vi "Kbd_Event_key_demo(copy).vi"() -> ()   [LabVIEW 2012]
panel:
  in  "error in":errorcluster
  out "error out":errorcluster
  in  "String":string="1234"
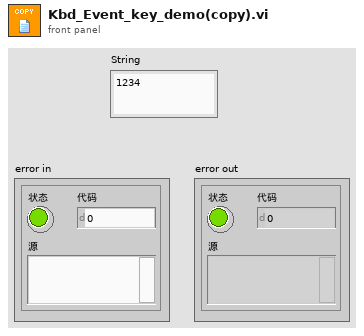
[diagram p1: front panel]
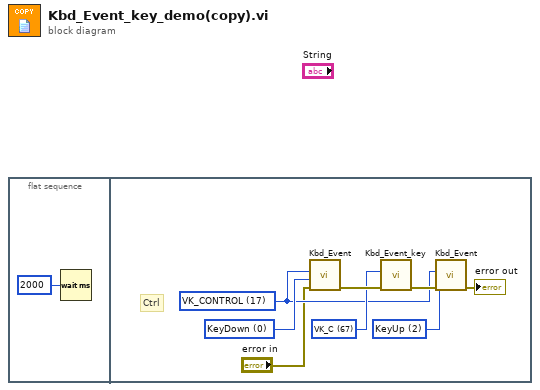
[diagram p0: block diagram]
diagram:
  n1 = flat-sequence {
    frame #0 {
      n2 = Wait (ms)(milliseconds to wait=u32 2000) -> ()  [unwired: 1 out]
    }
    frame #1 {
      w7 = u8 67 items=["Undefined", "VK_LBUTTON", "VK_RBUTTON", "VK_CANCEL", "VK_MBUTTON", "VK_XBUTTON1", "VK_XBUTTON2", "Undefined", "VK_BACK", "VK_TAB", "Reserved", "Reserved", "VK_CLEAR", "VK_RETURN", "Undefined", "Undefined", "VK_SHIFT", "VK_CONTROL", "VK_MENU", "VK_PAUSE", "VK_CAPITAL", "VK_KANA", "Undefined", "VK_JUNJA", "VK_FINAL", "VK_HANJA", "Undefined", "VK_ESCAPE", "VK_CONVERT", "VK_NONCONVERT", "VK_ACCEPT", "VK_MODECHANGE", "VK_SPACE", "VK_PRIOR", "VK_NEXT", "VK_END", "VK_HOME", "VK_LEFT", "VK_UP", "VK_RIGHT", "VK_DOWN", "VK_SELECT", "VK_PRINT", "VK_EXECUTE", "VK_SNAPSHOT", "VK_INSERT", "VK_DELETE", "VK_HELP", "VK_0", "VK_1", "VK_2", "VK_3", "VK_4", "VK_5", "VK_6", "VK_7", "VK_8", "VK_9", "Undefined", "Undefined", "Undefined", "Undefined", "Undefined", "Undefined", "Undefined", "VK_A", "VK_B", "VK_C", "VK_D", "VK_E", "VK_F", "VK_G", "VK_H", "VK_I", "VK_J", "VK_K", "VK_L", "VK_M", "VK_N", "VK_O", "VK_P", "VK_Q", "VK_R", "VK_S", "VK_T", "VK_U", "VK_V", "VK_W", "VK_X", "VK_Y", "VK_Z", "VK_LWIN", "VK_RWIN", "VK_APPS", "Reserved", "VK_SLEEP", "VK_NUMPAD0", "VK_NUMPAD1", "VK_NUMPAD2", "VK_NUMPAD3", "VK_NUMPAD4", "VK_NUMPAD5", "VK_NUMPAD6", "VK_NUMPAD7", "VK_NUMPAD8", "VK_NUMPAD9", "VK_MULTIPLY", "VK_ADD", "VK_SEPARATOR", "VK_SUBTRACT", "VK_DECIMAL", "VK_DIVIDE", "VK_F1", "VK_F2", "VK_F3", "VK_F4", "VK_F5", "VK_F6", "VK_F7", "VK_F8", "VK_F9", "VK_F10", "VK_F11", "VK_F12", "VK_F13", "VK_F14", "VK_F15", "VK_F16", "VK_F17", "VK_F18", "VK_F19  ", "VK_F20 ", "VK_F21", "VK_F22 ", "VK_F23", "VK_F24", "Unsigned", "Unsigned", "Unsigned", "Unsigned", "Unsigned", "Unsigned", "Unsigned", "Unsigned", "VK_NUMLOCK", "VK_SCROLL", "OEM Specific", " OEM Speicfic", "OEM Speicfic", "OEM Specific", "OEM Specific", "Unassigned", "Unassigned", "Unassigned", "Unassigned", "Unassigned", "Unassigned", "Unassigned", "Unassigned", "Unassigned", "VK_LSHIFT", "VK_RSHIFT", "VK_LCONTROL", "VK_RCONTROL", "VK_LMENU", "VK_RMENU", "VK_BROWSER_BACK", "VK_BROWSER_FORWARD", "VK_BROWSER_REFRESH", "VK_BROWSER_STOP", "VK_BROWSER_SEARCH", "VK_BROWSER_FAVORITES ", "VK_BROWSER_HOME", "VK_VOLUME_MUTE", "VK_VOLUME_DOWN", "VK_VOLUME_UP", "VK_MEDIA_NEXT_TRACK", "VK_MEDIA_PREV_TRACK", "VK_MEDIA_STOP ", "VK_MEDIA_PLAY_PAUSE", "VK_LAUNCH_MAIL", "VK_LAUNCH_MEDIA_SELECT", "VK_LAUNCH_APP1", "VK_LAUNCH_APP2", "Reserved", "Reserved", "VK_OEM_1(;:)", "VK_OEM_PLUS(+) ", "VK_OEM_COMMA(,)", "VK_OEM_MINUS(-)", "VK_OEM_PERIOD(.)", "VK_OEM_2(/?)", "VK_OEM_3(~`)", "Reserved", "Reserved", "Reserved", "Reserved", "Reserved", "Reserved", "Reserved", "Reserved", "Reserved", "Reserved", "Reserved", "Reserved", "Reserved", "Reserved", "Reserved", "Reserved", "Reserved", "Reserved", "Reserved", "Reserved", "Reserved", "Reserved", "Reserved", "Reserved", "Reserved", "Reserved", "VK_OEM_4 ([{)", "VK_OEM_5 (\\|)", "VK_OEM_6 (]})", "VK_OEM_7 ('\")", "VK_OEM_8", "Reserved", "Reserved", "VK_OEM_102", "OEM Specific", "OEM Specific", "VK_PROCESSKEY", "OEM Specific", "VK_PACKET", "Unassigned", "OEM Specific", "OEM Specific", "OEM Specific", "OEM Specific", "OEM Specific", "OEM Specific", "OEM Specific", "OEM Specific", "OEM Specific", "OEM Specific", "OEM Specific", "OEM Specific", "OEM Specific", "VK_ATTN", "VK_CRSEL", "VK_EXSEL", "VK_EREOF", "VK_PLAY", "VK_ZOOM", "VK_NONAME", "VK_PA1", "VK_OEM_CLEAR "] ("VK_CODE 2")
      w5 = u8 17 items=["Undefined", "VK_LBUTTON", "VK_RBUTTON", "VK_CANCEL", "VK_MBUTTON", "VK_XBUTTON1", "VK_XBUTTON2", "Undefined", "VK_BACK", "VK_TAB", "Reserved", "Reserved", "VK_CLEAR", "VK_RETURN", "Undefined", "Undefined", "VK_SHIFT", "VK_CONTROL", "VK_MENU", "VK_PAUSE", "VK_CAPITAL", "VK_KANA", "Undefined", "VK_JUNJA", "VK_FINAL", "VK_HANJA", "Undefined", "VK_ESCAPE", "VK_CONVERT", "VK_NONCONVERT", "VK_ACCEPT", "VK_MODECHANGE", "VK_SPACE", "VK_PRIOR", "VK_NEXT", "VK_END", "VK_HOME", "VK_LEFT", "VK_UP", "VK_RIGHT", "VK_DOWN", "VK_SELECT", "VK_PRINT", "VK_EXECUTE", "VK_SNAPSHOT", "VK_INSERT", "VK_DELETE", "VK_HELP", "VK_0", "VK_1", "VK_2", "VK_3", "VK_4", "VK_5", "VK_6", "VK_7", "VK_8", "VK_9", "Undefined", "Undefined", "Undefined", "Undefined", "Undefined", "Undefined", "Undefined", "VK_A", "VK_B", "VK_C", "VK_D", "VK_E", "VK_F", "VK_G", "VK_H", "VK_I", "VK_J", "VK_K", "VK_L", "VK_M", "VK_N", "VK_O", "VK_P", "VK_Q", "VK_R", "VK_S", "VK_T", "VK_U", "VK_V", "VK_W", "VK_X", "VK_Y", "VK_Z", "VK_LWIN", "VK_RWIN", "VK_APPS", "Reserved", "VK_SLEEP", "VK_NUMPAD0", "VK_NUMPAD1", "VK_NUMPAD2", "VK_NUMPAD3", "VK_NUMPAD4", "VK_NUMPAD5", "VK_NUMPAD6", "VK_NUMPAD7", "VK_NUMPAD8", "VK_NUMPAD9", "VK_MULTIPLY", "VK_ADD", "VK_SEPARATOR", "VK_SUBTRACT", "VK_DECIMAL", "VK_DIVIDE", "VK_F1", "VK_F2", "VK_F3", "VK_F4", "VK_F5", "VK_F6", "VK_F7", "VK_F8", "VK_F9", "VK_F10", "VK_F11", "VK_F12", "VK_F13", "VK_F14", "VK_F15", "VK_F16", "VK_F17", "VK_F18", "VK_F19  ", "VK_F20 ", "VK_F21", "VK_F22 ", "VK_F23", "VK_F24", "Unsigned", "Unsigned", "Unsigned", "Unsigned", "Unsigned", "Unsigned", "Unsigned", "Unsigned", "VK_NUMLOCK", "VK_SCROLL", "OEM Specific", " OEM Speicfic", "OEM Speicfic", "OEM Specific", "OEM Specific", "Unassigned", "Unassigned", "Unassigned", "Unassigned", "Unassigned", "Unassigned", "Unassigned", "Unassigned", "Unassigned", "VK_LSHIFT", "VK_RSHIFT", "VK_LCONTROL", "VK_RCONTROL", "VK_LMENU", "VK_RMENU", "VK_BROWSER_BACK", "VK_BROWSER_FORWARD", "VK_BROWSER_REFRESH", "VK_BROWSER_STOP", "VK_BROWSER_SEARCH", "VK_BROWSER_FAVORITES ", "VK_BROWSER_HOME", "VK_VOLUME_MUTE", "VK_VOLUME_DOWN", "VK_VOLUME_UP", "VK_MEDIA_NEXT_TRACK", "VK_MEDIA_PREV_TRACK", "VK_MEDIA_STOP ", "VK_MEDIA_PLAY_PAUSE", "VK_LAUNCH_MAIL", "VK_LAUNCH_MEDIA_SELECT", "VK_LAUNCH_APP1", "VK_LAUNCH_APP2", "Reserved", "Reserved", "VK_OEM_1(;:)", "VK_OEM_PLUS(+) ", "VK_OEM_COMMA(,)", "VK_OEM_MINUS(-)", "VK_OEM_PERIOD(.)", "VK_OEM_2(/?)", "VK_OEM_3(~`)", "Reserved", "Reserved", "Reserved", "Reserved", "Reserved", "Reserved", "Reserved", "Reserved", "Reserved", "Reserved", "Reserved", "Reserved", "Reserved", "Reserved", "Reserved", "Reserved", "Reserved", "Reserved", "Reserved", "Reserved", "Reserved", "Reserved", "Reserved", "Reserved", "Reserved", "Reserved", "VK_OEM_4 ([{)", "VK_OEM_5 (\\|)", "VK_OEM_6 (]})", "VK_OEM_7 ('\")", "VK_OEM_8", "Reserved", "Reserved", "VK_OEM_102", "OEM Specific", "OEM Specific", "VK_PROCESSKEY", "OEM Specific", "VK_PACKET", "Unassigned", "OEM Specific", "OEM Specific", "OEM Specific", "OEM Specific", "OEM Specific", "OEM Specific", "OEM Specific", "OEM Specific", "OEM Specific", "OEM Specific", "OEM Specific", "OEM Specific", "OEM Specific", "VK_ATTN", "VK_CRSEL", "VK_EXSEL", "VK_EREOF", "VK_PLAY", "VK_ZOOM", "VK_NONAME", "VK_PA1", "VK_OEM_CLEAR "] ("VK_CODE")
      w4 = u32 2 items=["KeyDown"=0, "KeyUp"=2] ("Option")
      w9 = u32 0 items=["KeyDown"=0, "KeyUp"=2] ("Option")
      # "Ctrl"
      n3 = call "Kbd_Event.vi"("error in"="error in", "Option"=w9, "VK_CODE"=w5) -> ("error out"=w8:errorcluster)  [unwired: 8 in]
      n4 = call "Kbd_Event_key.vi"("error in"=w8, "VK_CODE"=w7) -> ("error out"=w6:errorcluster)  [unwired: 9 in]
      n5 = call "Kbd_Event.vi"("error in"=w6, "Option"=w4, "VK_CODE"=w5) -> ("error out"=→"error out":errorcluster)  [unwired: 8 in]
    }
  }
